vi "Scripting_AddVIBetweenVIs.vi"(0 "ViToModify":refnum<vi>, 1 "VIToAdd":path, 2 "VIOne(Path,Name or NamePattern)":variant, 3 "VITwo(Path,Name or NamePattern), If Left/Right-string, it will be placed to the right or left of VIOne":variant, 4 "KeepSubVINodeRefOpen(False)":bool, 5 "error in (no error)":errorcluster) -> (15 "SubVI Refnum":refnum<vi>, 19 "error out":errorcluster)   [LabVIEW 2016]
uses:
  <vilib>/Utility/miscctls.llb/LVPointTypeDef.ctl
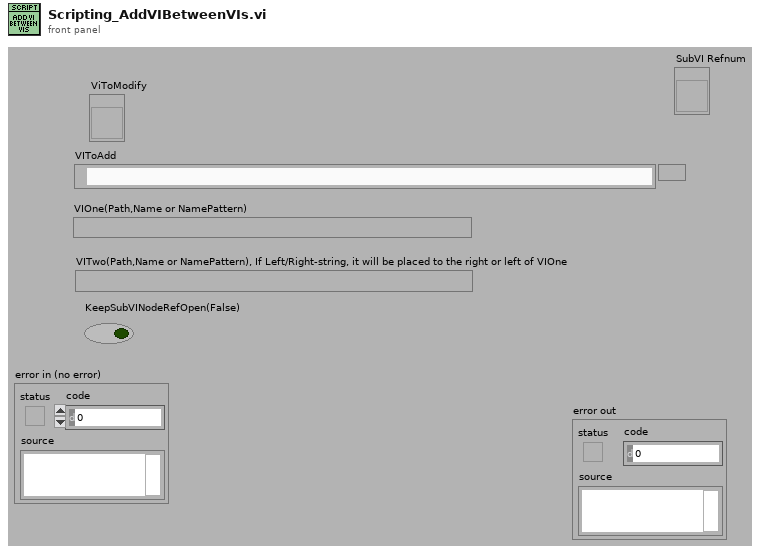
[diagram p1: front panel]
types:
  T1 = typedef "LVPointTypeDef.ctl" = cluster{"Horizontal":i16, "Vertical":i16}
  T2 = typedef "LVPositionTypeDef.ctl" = cluster{"Left":i32, "Top":i32}
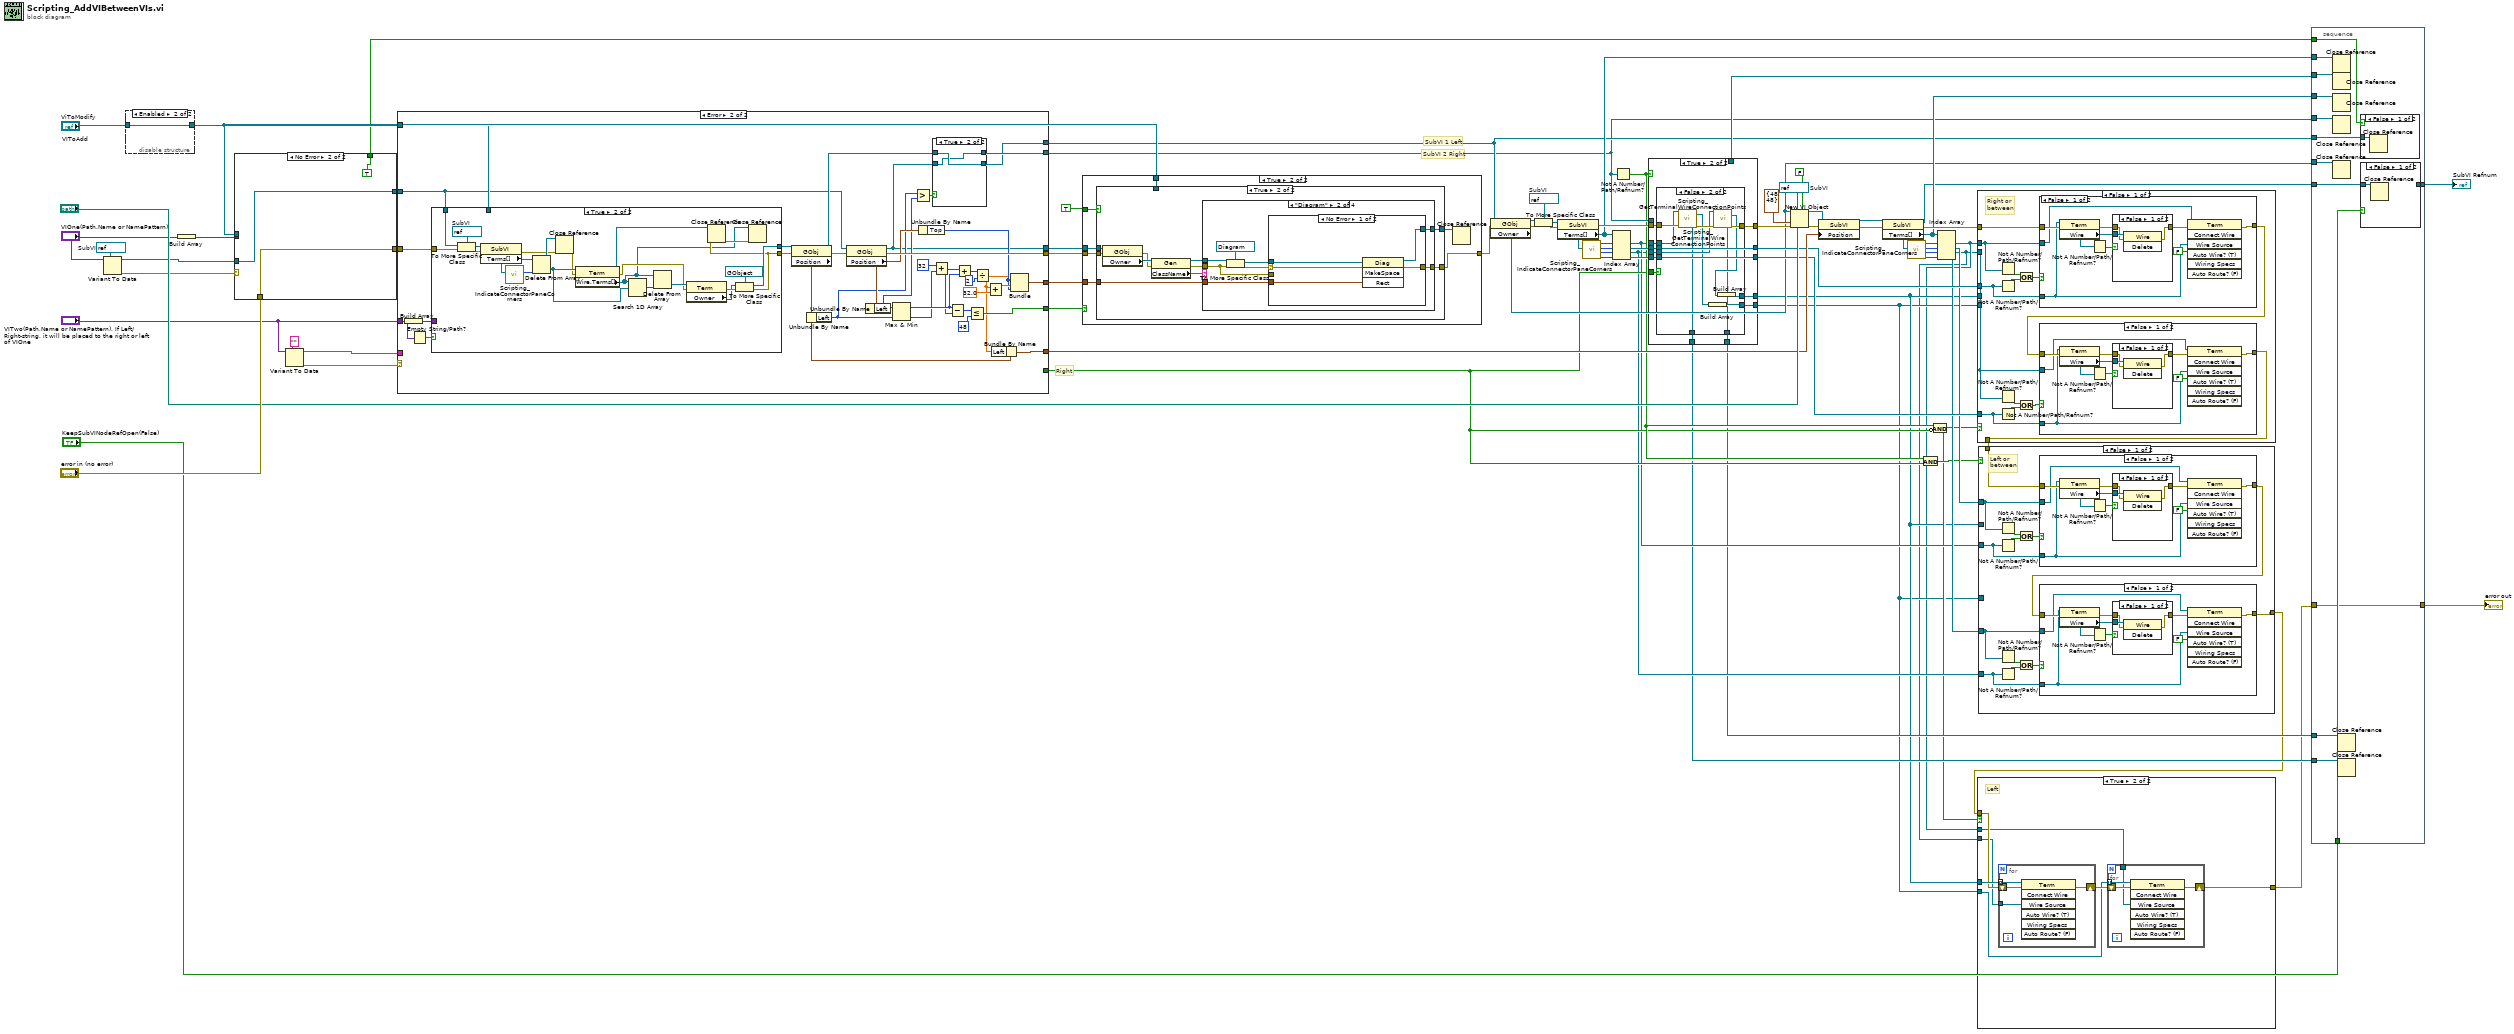
[diagram p0: block diagram]
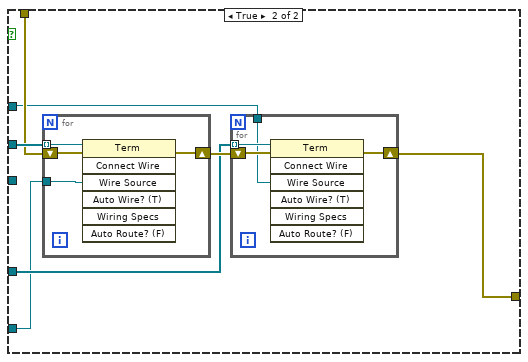
[diagram p7: hidden frame]
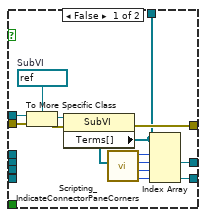
[diagram p13: hidden frame]
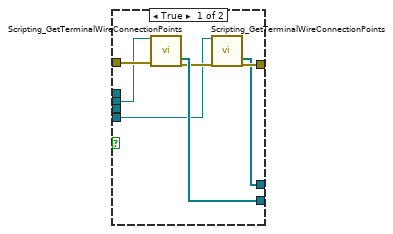
[diagram p14: hidden frame]
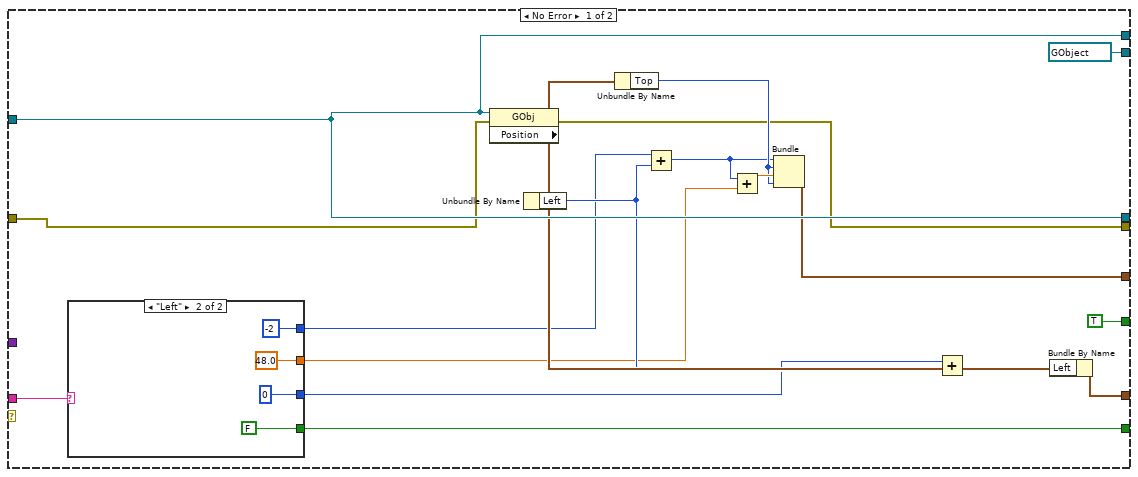
[diagram p15: hidden frame]
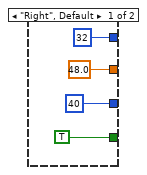
[diagram p16: hidden frame]
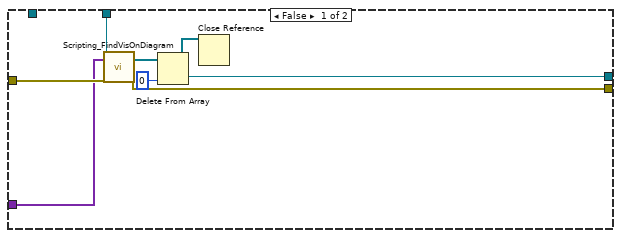
[diagram p17: hidden frame]
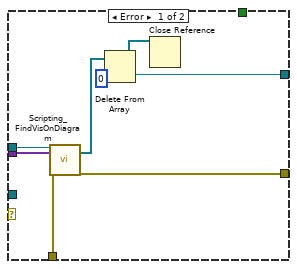
[diagram p19: hidden frame]
diagram:
  w29 = refnum<vi> refnum  # SubVI
  w52 = refnum<vi> refnum  # SubVI
  w77 = refnum<vi> refnum  # SubVI
  # "Right"
  # "SubVI 2 Right"
  # "SubVI 1 Left"
  n1 = Variant To Data(type=w29, Variant="VIOne(Path,Name or NamePattern)") -> (data=w27:refnum<vi>, error out=w28:errorcluster)  [unwired: 1 in]
  n2 = disable-structure shown="Enabled" {
    disable-tunnel: "ViToModify" -> [w80 w81]
    disable-tunnel: [w79 w81] -> w59
    frame Disabled {
      n3 = property class="VI"(reference=w80, "Front Panel.Open"=TRUE ("Front Panel Window:Open")) -> (reference out=w79:refnum<vi>)  [unwired: 1 in, 1 out]
    }
    frame Enabled {
    }
  }
  n4 = Build Array("VIOne(Path,Name or NamePattern)") -> (w66:variant[])
  n5 = case shown="No Error" w28 {
    tunnel: w66 -> [w89 _]
    tunnel: "error in (no error)" -> [w88 w91]
    tunnel: [w87 w91] -> w64
    tunnel: w59 -> [w83 _]
    tunnel: [w82 w92] -> w31
    tunnel: w27 -> [_ w92]
    tunnel: [_ TRUE] -> w1
    frame Error {
      n6 = call <resource>:"Scripting_FindVisOnDiagram.vi"("ViRef"=w83, "VIsToSerachFor/ViName"=w89, "error in (no error)"=w88) -> ("VisFound"=w86:refnum<vi>[], "error out"=w87:errorcluster)  [unwired: 15 in]
      n7 = Delete From Array(array=w86, index=0) -> (deleted portion=w82:refnum<vi>, array with subset deleted=w84:refnum<vi>[])  [unwired: 1 in]
      n8 = Close Reference(reference=w84) -> ()  [unwired: 1 in, 1 out]
    }
    frame No Error {
    }
  }
  n9 = Variant To Data(type="", Variant="VITwo(Path,Name or NamePattern), If Left/Right-string, it will be placed to the right or left of VIOne") -> (data=w19:string, error out=w23:errorcluster)  [unwired: 1 in]
  n10 = case shown="Error" w23 {
    tunnel: w64 -> [w105 w152]
    tunnel: [w104 w145] -> w62
    tunnel: [TRUE w144] -> w61
    tunnel: w59 -> [_ w143]
    tunnel: [w103 w134] -> w58
    tunnel: [w102 w131] -> w55
    tunnel: [w106 w126] -> w50
    tunnel: [refnum<vi> refnum ("WhileLoop") w125] -> w22
    tunnel: w31 -> [w106 w121]
    tunnel: [w106 w120] -> w26
    tunnel: "VITwo(Path,Name or NamePattern), If Left/Right-string, it will be placed to the right or left of VIOne" -> [_ w119]
    tunnel: w19 -> [w97 _]
    tunnel: [w96 _] -> w16
    frame No Error {
      n11 = case shown="\"Left\"" w97 {
        tunnel: [TRUE FALSE] -> w96
        tunnel: [32 ("x") -2 ("x")] -> w95
        tunnel: [48.0 ("y") 48.0 ("y")] -> w94
        tunnel: [40 ("x") 0 ("x")] -> w93
        frame "Right", Default {
        }
        frame "Left" {
        }
      }
      n12 = property class="GObj"(reference=w106, error in=w105) -> (error out=w104:errorcluster, "Position"=w101:T2)  [unwired: 1 out]
      n13 = Unbundle By Name(w101) -> ("Left"=w98:i32)
      n14 = Unbundle By Name(w101) -> ("Top"=w107:i32)
      n15 = Add(x=w95, y=w98) -> (x+y=w100:i32)
      n16 = Add(x=w100, y=w94) -> (x+y=w108:dbl)
      n17 = Bundle(w100, "Top"=w107, w108, "Top"=w107) -> (w103:cluster{i32, "Top":i32, dbl, "Top":i32})  [unwired: 1 in]
      n18 = Add(x=w93, y=w98) -> (x+y=w99:i32)
      n19 = Bundle By Name(cluster=w101, "Left"=w99) -> (w102:T2)
    }
    frame Error {
      n20 = Build Array(w119) -> (w151:variant[])
      n21 = Empty String/Path?(string/path=w119) -> (empty?=w122:bool)
      n22 = case shown="True" w122 {
        tunnel: w152 -> [w160 w178]
        tunnel: w151 -> [w159 _]
        tunnel: [w156 w168] -> w150
        tunnel: [w155 w164] -> w149
        tunnel: w143 -> [w154 _]
        tunnel: w121 -> [_ w180]
        frame False {
          n23 = call <resource>:"Scripting_FindVisOnDiagram.vi"("ViRef"=w154, "VIsToSerachFor/ViName"=w159, "error in (no error)"=w160) -> ("VisFound"=w158:refnum<vi>[], "error out"=w155:errorcluster)  [unwired: 15 in]
          n24 = Delete From Array(array=w158, index=0) -> (deleted portion=w156:refnum<vi>, array with subset deleted=w157:refnum<vi>[])  [unwired: 1 in]
          n25 = Close Reference(reference=w157) -> ()  [unwired: 1 in, 1 out]
        }
        frame True {
          w179 = refnum<vi> refnum  # SubVI
          n26 = To More Specific Class(target class=w179, reference=w180, error in=w178) -> (specific class reference=w182:refnum<vi>, error out=w181:errorcluster)
          n27 = property class="SubVI"(reference=w182, error in=w181) -> (error out=w166:errorcluster, "Terms[]"=w177:refnum<vi>[])  [unwired: 1 out]
          n28 = call <resource>:"Scripting_IndicateConnectorPaneCorners.vi"("Terminals[]"=w177) -> ("RightTop"=w176:i32)  [unwired: 7 in, 3 out]
          n29 = Delete From Array(array=w177, index=w176) -> (deleted portion=w174:refnum<vi>, array with subset deleted=w175:refnum<vi>[])  [unwired: 1 in]
          n30 = Close Reference(reference=w175, error in (no error)=w166) -> (error out=w165:errorcluster)
          n31 = property class="Term"(reference=w174, error in=w165) -> (reference out=w163:refnum<vi>, error out=w167:errorcluster, "Wire.Terms[]"=w161:refnum<vi>[])
          n32 = Search 1D Array(1D array=w161, element=w174) -> (index of element=w173:i32)  [unwired: 1 in]
          n33 = Delete From Array(array=w161, index=w173) -> (deleted portion=w172:refnum<vi>)  [unwired: 1 in, 1 out]
          n34 = property class="Term"(reference=w172, error in=w167) -> (error out=w171:errorcluster, "Owner"=w170:refnum<vi>)  [unwired: 1 out]
          n35 = To More Specific Class(target class=refnum<vi> refnum ("reference"), reference=w170, error in=w171) -> (specific class reference=w168:refnum<vi>, error out=w164:errorcluster)
          n36 = Close Reference(reference=w163, error in (no error)=w164) -> (error out=w162:errorcluster)
          n37 = Close Reference(reference=w161, error in (no error)=w162) -> ()  [unwired: 1 out]
        }
      }
      n38 = property class="GObj"(reference=w150, error in=w149) -> (reference out=w127:refnum<vi>, error out=w148:errorcluster, "Position"=w133:T2)
      n39 = Unbundle By Name(w133) -> ("Left"=w130:i32)
      n40 = property class="GObj"(reference=w121, error in=w148) -> (reference out=w126:refnum<vi>, error out=w145:errorcluster, "Position"=w136:T2)
      n41 = Unbundle By Name(w136) -> ("Left"=w129:i32)
      n42 = Max & Min(x=w129, y=w130) -> (max(x,y)=w140:i32, min(x,y)=w123:i32)
      n43 = Greater?(x=w130, y=w129) -> (0:w128:bool)
      n44 = Unbundle By Name(w136) -> ("Top"=w135:i32)
      n45 = case shown="True" w128 {
        tunnel: [w183 w186] -> w120
        tunnel: [w184 w185] -> w125
        tunnel: w127 -> [w184 w186]
        tunnel: w126 -> [w183 w185]
        frame False {
        }
        frame True {
        }
      }
      n46 = Add(x=32, y=w123) -> (x+y=w124:i32)
      n47 = Subtract(x=w140, y=w124) -> (x-y=w147:i32)
      n48 = Add(x=w124, y=w140) -> (x+y=w139:i32)
      n49 = Less Or Equal?(x=w147, y=48) -> (x <= y?=w144:bool)
      n50 = Divide(x=w139, y=2) -> (x/y=w132:dbl)
      n51 = Add(x=w132, y=32.0) -> (x+y=w137:dbl)
      n52 = Bundle By Name(cluster=w133, "Left"=w132) -> (w131:T2)
      n53 = Bundle(w132, "Top"=w135, w137, "Top"=w135) -> (w134:cluster{dbl, "Top":i32, dbl, "Top":i32})  [unwired: 1 in]
    }
  }
  n54 = case shown="True" w61 {
    tunnel: w50 -> [_ w194]
    tunnel: w62 -> [w187 w193]
    tunnel: TRUE -> [_ w192]
    tunnel: w59 -> [_ w191]
    tunnel: w58 -> [_ w190]
    tunnel: [w187 w189] -> w54
    frame False {
    }
    frame True {
      n55 = case shown="True" w192 {
        tunnel: w194 -> [_ w207]
        tunnel: w193 -> [w196 w206]
        tunnel: w191 -> [w200 _]
        tunnel: w190 -> [w199 w204]
        tunnel: [w198 w203] -> w189
        tunnel: [w195 w202] -> w188
        frame False {
          n56 = property class="VI"(reference=w200, error in=w196) -> (error out=w197:errorcluster, "Diagram"=w201:refnum<vi>)  [unwired: 1 out]
          n57 = invoke class="TopLvlDiag" method="MakeSpace"(reference=w201, error in=w197, "Rect"=w199) -> (reference out=w195:refnum<vi>, error out=w198:errorcluster)  [unwired: 1 in, 2 out]
        }
        frame True {
          n58 = property class="GObj"(reference=w207, error in=w206) -> (error out=w205:errorcluster, "Owner"=w208:refnum<vi>)  [unwired: 1 out]
          n59 = property class="Gen"(reference=w208, error in=w205) -> (reference out=w211:refnum<vi>, error out=w210:errorcluster, "ClassName"=w209:string)
          n60 = case shown="\"Diagram\"" w209 {
            tunnel: w211 -> [_ w219 w234 w249]
            tunnel: w210 -> [w212 w214 w229 w244]
            tunnel: w204 -> [_ w216 w231 w246]
            tunnel: [w212 w215 w230 w245] -> w203
            tunnel: [_ w213 w228 w243] -> w202
            frame Default {
            }
            frame "Diagram" {
              n61 = To More Specific Class(target class=refnum<vi> refnum ("Block Diagram"), reference=w219, error in=w214) -> (specific class reference=w217:refnum<vi>, error out=w220:errorcluster)
              n62 = case shown="No Error" w220 {
                selector: w220 -> [w225 _]
                tunnel: w217 -> [w224 w226]
                tunnel: w216 -> [w223 _]
                tunnel: [w222 w227] -> w215
                tunnel: w214 -> [_ w227]
                tunnel: [w221 w226] -> w213
                frame No Error {
                  n63 = invoke class="Diag" method="MakeSpace"(reference=w224, error in=w225, "Rect"=w223) -> (reference out=w221:refnum<vi>, error out=w222:errorcluster)  [unwired: 1 in, 2 out]
                }
                frame Error {
                }
              }
            }
            frame "TopLevelDiagram" {
              n64 = To More Specific Class(target class=refnum<vi> refnum ("Block Diagram"), reference=w234, error in=w229) -> (specific class reference=w232:refnum<vi>, error out=w235:errorcluster)
              n65 = case shown="No Error" w235 {
                selector: w235 -> [w240 _]
                tunnel: w232 -> [w239 w241]
                tunnel: w231 -> [w238 _]
                tunnel: [w237 w242] -> w230
                tunnel: w229 -> [_ w242]
                tunnel: [w236 w241] -> w228
                frame No Error {
                  n66 = invoke class="TopLvlDiag" method="MakeSpace"(reference=w239, error in=w240, "Rect"=w238) -> (reference out=w236:refnum<vi>, error out=w237:errorcluster)  [unwired: 1 in, 2 out]
                }
                frame Error {
                }
              }
            }
            frame "CaseStructure" {
              n67 = To More Specific Class(target class=refnum<vi> refnum ("Block Diagram"), reference=w249, error in=w244) -> (specific class reference=w248:refnum<vi>, error out=w250:errorcluster)
              n68 = case shown="Error" w250 {
                selector: w250 -> [w258 _]
                tunnel: w249 -> [w251 w260]
                tunnel: w248 -> [w259 _]
                tunnel: w246 -> [w253 _]
                tunnel: [w252 w261] -> w245
                tunnel: w244 -> [_ w261]
                tunnel: [w251 w260] -> w243
                frame No Error {
                  n69 = property class="CaseSel"(reference=w259, error in=w258) -> (error out=w256:errorcluster, "Diagrams"=w254:refnum<vi>[])  [unwired: 1 out]
                  n70 = Index Array(array=w254) -> (element=w257:refnum<vi>)  [unwired: 1 in]
                  n71 = invoke class="Diag" method="MakeSpace"(reference=w257, error in=w256, "Rect"=w253) -> (error out=w255:errorcluster)  [unwired: 1 in, 3 out]
                  n72 = Close Reference(reference=w254, error in (no error)=w255) -> (error out=w252:errorcluster)
                }
                frame Error {
                }
              }
            }
          }
        }
      }
      n73 = Close Reference(reference=w188) -> ()  [unwired: 1 in, 1 out]
    }
  }
  n74 = property class="GObj"(reference=w26, error in=w54) -> (reference out=w53:refnum<vi>, error out=w51:errorcluster, "Owner"=w32:refnum<vi>)
  n75 = To More Specific Class(target class=w52, reference=w53, error in=w51) -> (specific class reference=w45:refnum<vi>, error out=w44:errorcluster)
  n76 = property class="SubVI"(reference=w45, error in=w44) -> (error out=w43:errorcluster, "Terms[]"=w36:refnum<vi>[])  [unwired: 1 out]
  n77 = call <resource>:"Scripting_IndicateConnectorPaneCorners.vi"("Terminals[]"=w36) -> ("RightLower"=w49:i32, "LeftLower"=w48:i32, "RightTop"=w47:i32, "LeftTop"=w46:i32)  [unwired: 7 in]
  n78 = Index Array(array=w36, index #1=w46, index #2=w47, index #3=w48, index #4=w49) -> (element #1=w15:refnum<vi>, element #2=w20:refnum<vi>, element #3=w14:refnum<vi>, element #4=w21:refnum<vi>)
  n79 = Not A Number/Path/Refnum?(number/path/refnum=w22) -> (NaN/Path/Refnum?=w17:bool)
  n80 = case shown="True" w17 {
    tunnel: w43 -> [w267 w285]
    tunnel: [w266 w282] -> w42
    tunnel: [w265 w284] -> w41
    tunnel: [w264 w281] -> w39
    tunnel: [w263 _] -> w35
    tunnel: w22 -> [w262 _]
    tunnel: w21 -> [_ w281]
    tunnel: w20 -> [_ w284]
    tunnel: [_ w283] -> w7
    tunnel: [_ w280] -> w8
    tunnel: w16 -> [_ w279]
    tunnel: w15 -> [_ w278]
    tunnel: w14 -> [_ w277]
    tunnel: [_ w276] -> w13
    tunnel: [_ w275] -> w12
    frame False {
      w274 = refnum<vi> refnum  # SubVI
      n81 = To More Specific Class(target class=w274, reference=w262, error in=w267) -> (specific class reference=w269:refnum<vi>, error out=w268:errorcluster)
      n82 = property class="SubVI"(reference=w269, error in=w268) -> (error out=w266:errorcluster, "Terms[]"=w263:refnum<vi>[])  [unwired: 1 out]
      n83 = call <resource>:"Scripting_IndicateConnectorPaneCorners.vi"("Terminals[]"=w263) -> ("RightLower"=w270:i32, "LeftLower"=w271:i32, "RightTop"=w272:i32, "LeftTop"=w273:i32)  [unwired: 7 in]
      n84 = Index Array(array=w263, index #1=w273, index #2=w272, index #3=w271, index #4=w270) -> (element #2=w265:refnum<vi>, element #4=w264:refnum<vi>)  [unwired: 2 out]
    }
    frame True {
      n85 = case shown="False" w279 {
        tunnel: w285 -> [w292 w303]
        tunnel: w284 -> [w291 _]
        tunnel: [w290 w297] -> w283
        tunnel: [w288 w301] -> w282
        tunnel: w281 -> [w287 _]
        tunnel: [w286 w296] -> w280
        tunnel: w278 -> [_ w300]
        tunnel: w277 -> [_ w299]
        tunnel: [_ w294] -> w276
        tunnel: [_ w293] -> w275
        frame True {
          n86 = call <resource>:"Scripting_GetTerminalWireConnectionPoints.vi"("Term Refnum In"=w291, "error in"=w292) -> ("AllWireTerminalDrains"=w290:refnum<vi>[], "error out"=w289:errorcluster)  [unwired: 9 in, 7 out]
          n87 = call <resource>:"Scripting_GetTerminalWireConnectionPoints.vi"("Term Refnum In"=w287, "error in"=w289) -> ("AllWireTerminalDrains"=w286:refnum<vi>[], "error out"=w288:errorcluster)  [unwired: 9 in, 7 out]
        }
        frame False {
          n88 = call <resource>:"Scripting_GetTerminalWireConnectionPoints.vi"("Term Refnum In"=w300, "error in"=w303) -> ("AllWireTerminals"=w294:refnum<vi>[], "WireTermSource"=w298:refnum<vi>, "error out"=w302:errorcluster)  [unwired: 9 in, 6 out]
          n89 = Build Array(w298) -> (w297:refnum<vi>[])
          n90 = call <resource>:"Scripting_GetTerminalWireConnectionPoints.vi"("Term Refnum In"=w299, "error in"=w302) -> ("AllWireTerminals"=w293:refnum<vi>[], "WireTermSource"=w295:refnum<vi>, "error out"=w301:errorcluster)  [unwired: 9 in, 6 out]
          n91 = Build Array(w295) -> (w296:refnum<vi>[])
        }
      }
    }
  }
  n92 = New VI Object(vi object class=w77, auto wire? (F)=FALSE, owner refnum=w32, position/next to=T1 {"Horizontal"=48, "Vertical"=48} ("relative position/next to refnum"), 6:"VIToAdd", 8:w42) -> (object refnum=w74:refnum<vi>, 0:w75:errorcluster)  [unwired: 2 in]
  n93 = property class="SubVI"(reference=w74, error in=w75, "Position"=w55) -> (reference out=w56:refnum<vi>, error out=w57:errorcluster)
  n94 = property class="SubVI"(reference=w56, error in=w57) -> (reference out=w33:refnum<vi>, error out=w71:errorcluster, "Terms[]"=w34:refnum<vi>[])
  n95 = call <resource>:"Scripting_IndicateConnectorPaneCorners.vi"("Terminals[]"=w34) -> ("RightLower"=w69:i32, "LeftLower"=w70:i32, "RightTop"=w72:i32, "LeftTop"=w73:i32)  [unwired: 7 in]
  n96 = Compound Arithmetic op=AND(w17, w16) -> (w18:bool)
  n97 = Compound Arithmetic op=AND(w17, invert w16) -> (w9:bool)
  n98 = Index Array(array=w34, index #1=w73, index #2=w72, index #3=w70, index #4=w69) -> (element #1=w6:refnum<vi>, element #2=w38:refnum<vi>, element #3=w5:refnum<vi>, element #4=w37:refnum<vi>)
  n99 = case shown="False" w9 {
    tunnel: w71 -> [w316 w345]
    tunnel: w6 -> [w312 _]
    tunnel: w41 -> [w311 _]
    tunnel: [w307 w345] -> w40
    tunnel: w5 -> [w305 _]
    tunnel: w39 -> [w304 _]
    tunnel: w8 -> [_ _]
    tunnel: w7 -> [_ _]
    frame False {
      # "Right or\nbetween"
      n100 = Not A Number/Path/Refnum?(number/path/refnum=w312) -> (NaN/Path/Refnum?=w315:bool)
      n101 = Not A Number/Path/Refnum?(number/path/refnum=w311) -> (NaN/Path/Refnum?=w314:bool)
      n102 = Not A Number/Path/Refnum?(number/path/refnum=w305) -> (NaN/Path/Refnum?=w308:bool)
      n103 = Not A Number/Path/Refnum?(number/path/refnum=w304) -> (NaN/Path/Refnum?=w309:bool)
      n104 = Or(x=w315, y=w314) -> (x .or. y?=w313:bool)
      n105 = Or(x=w308, y=w309) -> (x .or. y?=w310:bool)
      n106 = case shown="False" w313 {
        tunnel: w316 -> [w337 w344]
        tunnel: [w339 w344] -> w306
        tunnel: w312 -> [w331 _]
        tunnel: w311 -> [w332 _]
        frame False {
          n107 = property class="Term"(reference=w332, error in=w337) -> (error out=w335:errorcluster, "Wire"=w336:refnum<vi>)  [unwired: 1 out]
          n108 = Not A Number/Path/Refnum?(number/path/refnum=w336) -> (NaN/Path/Refnum?=w334:bool)
          n109 = case shown="False" w334 {
            tunnel: [w342 w343] -> w338
            tunnel: w336 -> [w341 _]
            tunnel: w335 -> [w340 w343]
            frame False {
              n110 = invoke class="Wire" method="Delete"(reference=w341, error in=w340) -> (error out=w342:errorcluster)  [unwired: 1 in, 2 out]
            }
            frame True {
            }
          }
          n111 = invoke class="Term" method="Connect Wire"(reference=w331, error in=w338, "Wire Source"=w332, "Auto Wire? (T)"=FALSE) -> (error out=w339:errorcluster)  [unwired: 3 in, 6 out]
        }
        frame True {
        }
      }
      n112 = case shown="False" w310 {
        tunnel: w306 -> [w323 w330]
        tunnel: [w325 w330] -> w307
        tunnel: w305 -> [w318 _]
        tunnel: w304 -> [w317 _]
        frame False {
          n113 = property class="Term"(reference=w317, error in=w323) -> (error out=w321:errorcluster, "Wire"=w322:refnum<vi>)  [unwired: 1 out]
          n114 = Not A Number/Path/Refnum?(number/path/refnum=w322) -> (NaN/Path/Refnum?=w320:bool)
          n115 = case shown="False" w320 {
            tunnel: [w328 w329] -> w324
            tunnel: w322 -> [w327 _]
            tunnel: w321 -> [w326 w329]
            frame False {
              n116 = invoke class="Wire" method="Delete"(reference=w327, error in=w326) -> (error out=w328:errorcluster)  [unwired: 1 in, 2 out]
            }
            frame True {
            }
          }
          n117 = invoke class="Term" method="Connect Wire"(reference=w318, error in=w324, "Wire Source"=w317, "Auto Wire? (T)"=FALSE) -> (error out=w325:errorcluster)  [unwired: 3 in, 6 out]
        }
        frame True {
        }
      }
    }
    frame True {
      # "Left"
    }
  }
  n118 = case shown="False" w18 {
    tunnel: w40 -> [w351 w390]
    tunnel: [w350 w389] -> w11
    tunnel: w38 -> [w349 w388]
    tunnel: w15 -> [w348 _]
    tunnel: w37 -> [w347 w387]
    tunnel: w14 -> [w346 _]
    tunnel: w8 -> [_ w393]
    tunnel: w7 -> [_ w391]
    frame False {
      # "Left or\nbetween"
      n119 = Not A Number/Path/Refnum?(number/path/refnum=w349) -> (NaN/Path/Refnum?=w358:bool)
      n120 = Not A Number/Path/Refnum?(number/path/refnum=w348) -> (NaN/Path/Refnum?=w357:bool)
      n121 = Not A Number/Path/Refnum?(number/path/refnum=w347) -> (NaN/Path/Refnum?=w353:bool)
      n122 = Not A Number/Path/Refnum?(number/path/refnum=w346) -> (NaN/Path/Refnum?=w354:bool)
      n123 = Or(x=w358, y=w357) -> (x .or. y?=w356:bool)
      n124 = Or(x=w353, y=w354) -> (x .or. y?=w355:bool)
      n125 = case shown="False" w356 {
        tunnel: w351 -> [w379 w386]
        tunnel: [w381 w386] -> w352
        tunnel: w349 -> [w374 _]
        tunnel: w348 -> [w373 _]
        frame False {
          n126 = property class="Term"(reference=w373, error in=w379) -> (error out=w377:errorcluster, "Wire"=w378:refnum<vi>)  [unwired: 1 out]
          n127 = Not A Number/Path/Refnum?(number/path/refnum=w378) -> (NaN/Path/Refnum?=w376:bool)
          n128 = case shown="False" w376 {
            tunnel: [w384 w385] -> w380
            tunnel: w378 -> [w383 _]
            tunnel: w377 -> [w382 w385]
            frame False {
              n129 = invoke class="Wire" method="Delete"(reference=w383, error in=w382) -> (error out=w384:errorcluster)  [unwired: 1 in, 2 out]
            }
            frame True {
            }
          }
          n130 = invoke class="Term" method="Connect Wire"(reference=w374, error in=w380, "Wire Source"=w373, "Auto Wire? (T)"=FALSE) -> (error out=w381:errorcluster)  [unwired: 3 in, 6 out]
        }
        frame True {
        }
      }
      n131 = case shown="False" w355 {
        tunnel: w352 -> [w365 w372]
        tunnel: [w367 w372] -> w350
        tunnel: w347 -> [w360 _]
        tunnel: w346 -> [w359 _]
        frame False {
          n132 = property class="Term"(reference=w359, error in=w365) -> (error out=w363:errorcluster, "Wire"=w364:refnum<vi>)  [unwired: 1 out]
          n133 = Not A Number/Path/Refnum?(number/path/refnum=w364) -> (NaN/Path/Refnum?=w362:bool)
          n134 = case shown="False" w362 {
            tunnel: [w370 w371] -> w366
            tunnel: w364 -> [w369 _]
            tunnel: w363 -> [w368 w371]
            frame False {
              n135 = invoke class="Wire" method="Delete"(reference=w369, error in=w368) -> (error out=w370:errorcluster)  [unwired: 1 in, 2 out]
            }
            frame True {
            }
          }
          n136 = invoke class="Term" method="Connect Wire"(reference=w360, error in=w366, "Wire Source"=w359, "Auto Wire? (T)"=FALSE) -> (error out=w367:errorcluster)  [unwired: 3 in, 6 out]
        }
        frame True {
        }
      }
    }
    frame True {
      n137 = for {
        tunnel: w393 -> [w401] mode=indexing
        shift-right: [w399] -> w392
        shift-left: w390 -> [w400]
        tunnel: w387 -> [w398]
        n138 = invoke class="Term" method="Connect Wire"(reference=w401, error in=w400, "Wire Source"=w398) -> (error out=w399:errorcluster)  [unwired: 4 in, 6 out]
      }
      n139 = for {
        tunnel: w391 -> [w397] mode=indexing
        shift-right: [w395] -> w389
        shift-left: w392 -> [w396]
        tunnel: w388 -> [w394]
        n140 = invoke class="Term" method="Connect Wire"(reference=w397, error in=w396, "Wire Source"=w394) -> (error out=w395:errorcluster)  [unwired: 4 in, 6 out]
      }
    }
  }
  n141 = case shown="True" w9 {
    tunnel: w11 -> [w402 w406]
    tunnel: w6 -> [_ w405]
    tunnel: [w402 w403] -> w10
    tunnel: w5 -> [_ w404]
    tunnel: w8 -> [_ w408]
    tunnel: w7 -> [_ w407]
    frame False {
      # "Right or\nbetween"
    }
    frame True {
      # "Left"
      n142 = for {
        tunnel: w408 -> [w417] mode=indexing
        shift-right: [w415] -> w409
        shift-left: w406 -> [w416]
        tunnel: w404 -> [w414]
        n143 = invoke class="Term" method="Connect Wire"(reference=w417, error in=w416, "Wire Source"=w414) -> (error out=w415:errorcluster)  [unwired: 4 in, 6 out]
      }
      n144 = for {
        tunnel: w407 -> [w413] mode=indexing
        shift-right: [w411] -> w403
        shift-left: w409 -> [w412]
        tunnel: w405 -> [w410]
        n145 = invoke class="Term" method="Connect Wire"(reference=w413, error in=w412, "Wire Source"=w410) -> (error out=w411:errorcluster)  [unwired: 4 in, 6 out]
      }
    }
  }
  n146 = stacked-sequence {
    tunnel: w10 -> [w420]
    tunnel: w36 -> [w430]
    tunnel: w35 -> [w429]
    tunnel: w34 -> [w428]
    tunnel: w33 -> [w427]
    tunnel: w22 -> [w426]
    tunnel: w26 -> [w425]
    tunnel: w32 -> [w424]
    tunnel: w13 -> [w423]
    tunnel: w12 -> [w422]
    tunnel: "KeepSubVINodeRefOpen(False)" -> [w421]
    tunnel: [w420] -> w3
    tunnel: [w419] -> w2
    tunnel: w1 -> [w418]
    frame #0 {
      n147 = Close Reference(reference=w430) -> ()  [unwired: 1 in, 1 out]
      n148 = Close Reference(reference=w429) -> ()  [unwired: 1 in, 1 out]
      n149 = Close Reference(reference=w428) -> ()  [unwired: 1 in, 1 out]
      n150 = Close Reference(reference=w426) -> ()  [unwired: 1 in, 1 out]
      n151 = Close Reference(reference=w424) -> ()  [unwired: 1 in, 1 out]
      n152 = Close Reference(reference=w422) -> ()  [unwired: 1 in, 1 out]
      n153 = Close Reference(reference=w423) -> ()  [unwired: 1 in, 1 out]
      n154 = case shown="False" w418 {
        tunnel: w425 -> [w431 _]
        frame False {
          n155 = Close Reference(reference=w431) -> ()  [unwired: 1 in, 1 out]
        }
        frame True {
        }
      }
      n156 = case shown="False" w421 {
        tunnel: w427 -> [w432 w433]
        tunnel: [_ w433] -> w419
        frame False {
          n157 = Close Reference(reference=w432) -> ()  [unwired: 1 in, 1 out]
        }
        frame True {
        }
      }
    }
  }
  "error out" <- w3
  "SubVI Refnum" <- w2
